vi "Display.vi"(10 "Case Selector":T2(ring)) -> (2 "Cluster":T1)   [LabVIEW 2016]
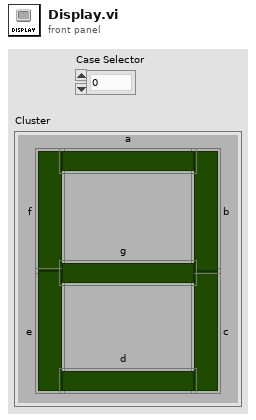
[diagram p1: front panel]
types:
  T1 = cluster{"f":bool, "e":bool, "c":bool, "b":bool, "d":bool, "g":bool, "a":bool}
  T2 = enum16{"0", "1", "2", "3", "4", "5", "6", "7", "8", "9"}
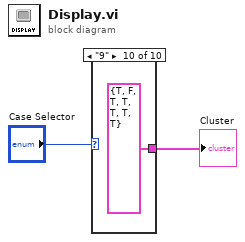
[diagram p0: block diagram]
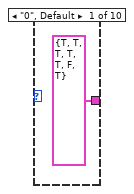
[diagram p2: hidden frame]
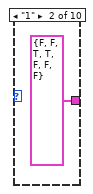
[diagram p3: hidden frame]
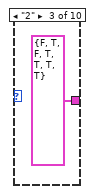
[diagram p4: hidden frame]
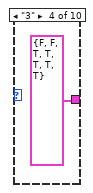
[diagram p5: hidden frame]
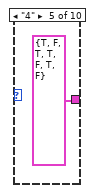
[diagram p6: hidden frame]
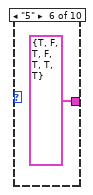
[diagram p7: hidden frame]
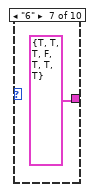
[diagram p8: hidden frame]
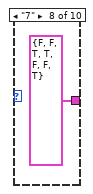
[diagram p9: hidden frame]
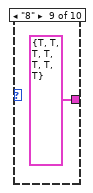
[diagram p10: hidden frame]
diagram:
  n1 = case shown="\"9\"" "Case Selector" {
    tunnel: [T1 {"f"=TRUE, "e"=TRUE, "c"=TRUE, "b"=TRUE, "d"=TRUE, "g"=FALSE, "a"=TRUE} ("Cluster 2") T1 {"f"=FALSE, "e"=FALSE, "c"=TRUE, "b"=TRUE, "d"=FALSE, "g"=FALSE, "a"=FALSE} ("Cluster 2") T1 {"f"=FALSE, "e"=TRUE, "c"=FALSE, "b"=TRUE, "d"=TRUE, "g"=TRUE, "a"=TRUE} ("Cluster 2") T1 {"f"=FALSE, "e"=FALSE, "c"=TRUE, "b"=TRUE, "d"=TRUE, "g"=TRUE, "a"=TRUE} ("Cluster 2") T1 {"f"=TRUE, "e"=FALSE, "c"=TRUE, "b"=TRUE, "d"=FALSE, "g"=TRUE, "a"=FALSE} ("Cluster 2") T1 {"f"=TRUE, "e"=FALSE, "c"=TRUE, "b"=FALSE, "d"=TRUE, "g"=TRUE, "a"=TRUE} ("Cluster 2") T1 {"f"=TRUE, "e"=TRUE, "c"=TRUE, "b"=FALSE, "d"=TRUE, "g"=TRUE, "a"=TRUE} ("Cluster 2") T1 {"f"=FALSE, "e"=FALSE, "c"=TRUE, "b"=TRUE, "d"=FALSE, "g"=FALSE, "a"=TRUE} ("Cluster 2") T1 {"f"=TRUE, "e"=TRUE, "c"=TRUE, "b"=TRUE, "d"=TRUE, "g"=TRUE, "a"=TRUE} ("Cluster 2") T1 {"f"=TRUE, "e"=FALSE, "c"=TRUE, "b"=TRUE, "d"=TRUE, "g"=TRUE, "a"=TRUE} ("Cluster 2")] -> w1
    frame "0", Default {
    }
    frame "1" {
    }
    frame "2" {
    }
    frame "3" {
    }
    frame "4" {
    }
    frame "5" {
    }
    frame "6" {
    }
    frame "7" {
    }
    frame "8" {
    }
    frame "9" {
    }
  }
  "Cluster" <- w1
